vi "test doublepush move.vi"() -> ()   [LabVIEW 2016]
uses:
  Chesslib/Position/Position.lvclass
  Chesslib/typedef/Piece.ctl
  Chesslib/typedef/Color.ctl
  Chesslib/typedef/Piece type.ctl
  Chesslib/typedef/Square.ctl
  Chesslib/typedef/File.ctl
  Chesslib/typedef/Rank.ctl
  Chesslib/Position/Position.lvclass/Position.ctl
  Chesslib/Chesslib.lvlib
  Chesslib/Board/Board.lvclass
  Chesslib/Moves/Move/Move.lvclass
panel:
  out "Valid move":bool
  out "Board layout":cluster{"Occupied":bool, "Piece":T1}[][](array[cluster])
  out "Position out":refnum<class "Position.lvclass">
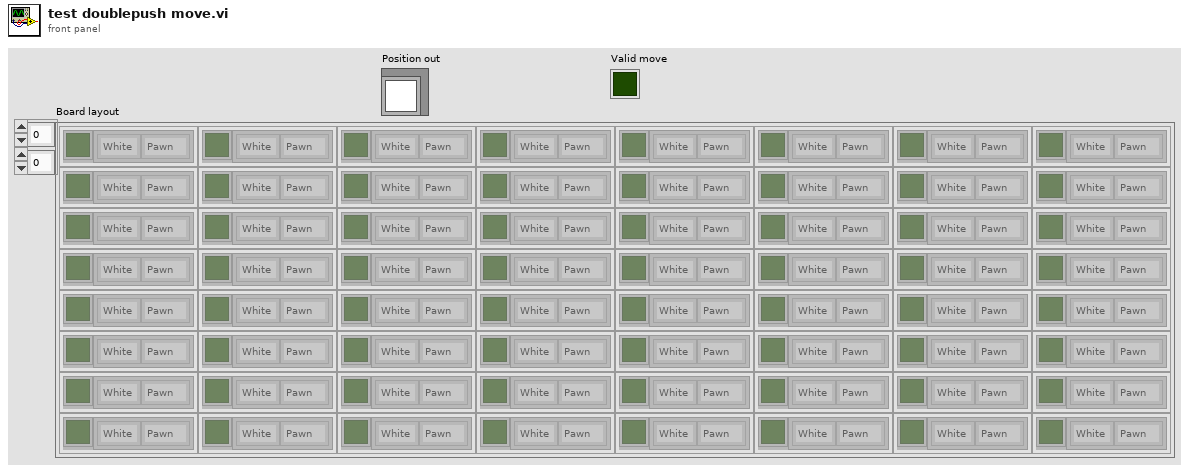
[diagram p1: front panel]
types:
  T1 = typedef "Chesslib.lvlib/Piece.ctl" = cluster{"Color":T2, "Type":T3}
  T2 = typedef "Chesslib.lvlib/Color.ctl" = enum16{"White", "Black"}
  T3 = typedef "Chesslib.lvlib/Piece type.ctl" = enum16{"Pawn", "Bishop", "Knight", "Rook", "Queen", "King"}
  T4 = typedef "Chesslib.lvlib/Square.ctl" = cluster{"File":T5, "Rank":T6}
  T5 = typedef "Chesslib.lvlib/File.ctl" = enum8{"a", "b", "c", "d", "e", "f", "g", "h"}
  T6 = typedef "Chesslib.lvlib/Rank.ctl" = enum8{"1", "2", "3", "4", "5", "6", "7", "8"}
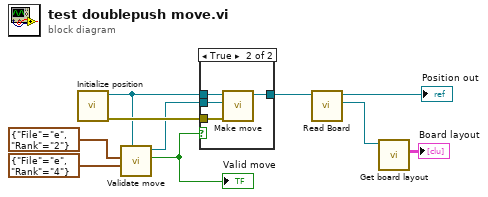
[diagram p0: block diagram]
diagram:
  n1 = call "Initialize position.vi"() -> ("error out"=w9:errorcluster, "Position out"=w3:refnum<class "Position.lvclass">)  [unwired: 10 in]
  n2 = call "Validate move.vi"("Position"=w3, "Destination"=T4 {"File"=enum."e", "Rank"=enum."4"}, "Source"=T4 {"File"=enum."e", "Rank"=enum."2"}) -> ("Valid move"=w1:bool, "Move"=w2:refnum<class "Move.lvclass">)  [unwired: 7 in]
  "Valid move" <- w1
  n3 = case shown="True" w1 {
    tunnel: [w11 w15] -> w10
    tunnel: w9 -> [_ w14]
    tunnel: w3 -> [w11 w13]
    tunnel: w2 -> [_ w12]
    frame False {
    }
    frame True {
      n4 = call "Make move.vi"("error in (no error)"=w14, "Move"=w12, "Position in"=w13) -> ("Position out"=w15:refnum<class "Position.lvclass">)  [unwired: 7 in, 1 out]
    }
  }
  n5 = call "Read Board.vi"("Position in"=w10) -> ("Board"=w7:refnum<class "Board.lvclass">, "Position out"=→"Position out":refnum<class "Position.lvclass">)  [unwired: 9 in]
  n6 = call "Get board layout.vi"("Board in"=w7) -> ("Board layout"=→"Board layout":cluster{"Occupied":bool, "Piece":T1}[][])  [unwired: 9 in, 1 out]
